vi "全局变量.vi"() -> ()   [LabVIEW 2011]
panel:
  in  "Gradient_Flag":bool
  in  "Overflow_Counter":u16
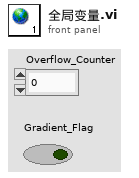
[diagram p1: front panel]
diagram:
